vi "Main Engine Path and Folder Info.vi"(8 "error in":errorcluster) -> (0 "error out":errorcluster, 1 "LabVIEW Data":path, 2 "Spare 2":path, 3 "Config":path, 4 "DynData File":path, 5 "Data Logging":path, 7 "TDMS-Logging":path)   [LabVIEW 2024]
doc: "All Rights Reserved © 2017 SyncSols"
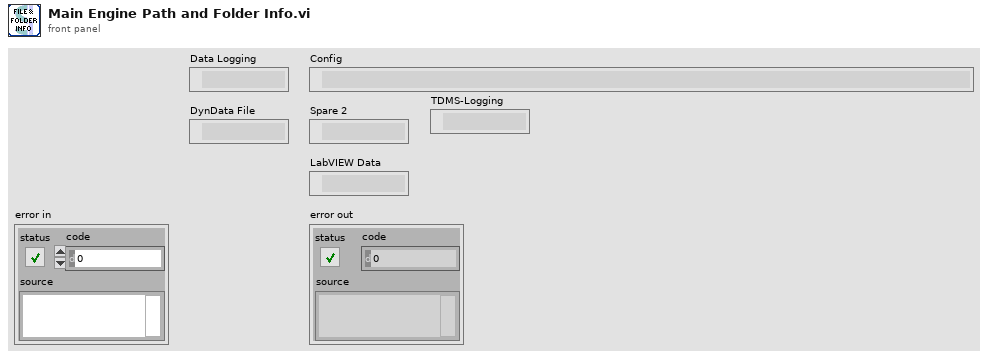
[diagram p1: front panel]
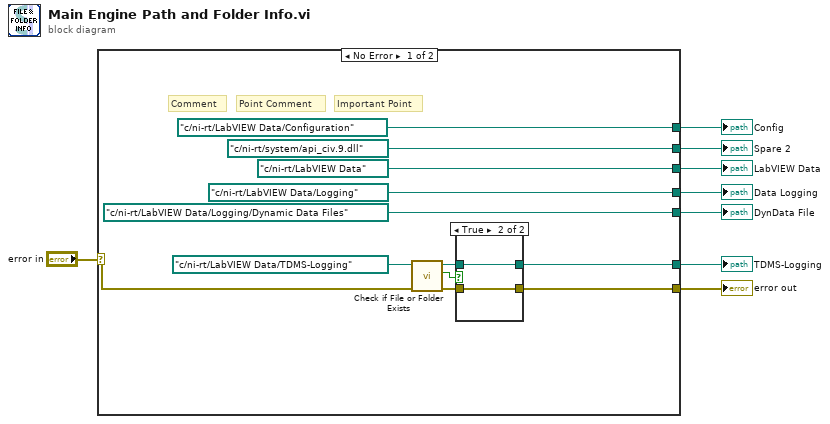
[diagram p0: block diagram]
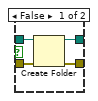
[diagram p2: hidden frame]
diagram:
  n1 = case shown="No Error" "error in" {
    selector: "error in" -> [w14 w27]
    tunnel: [w9 w27] -> w8
    tunnel: [path "c:/ni-rt/LabVIEW Data/Configuration" ("MIL 1553 B") _] -> w6
    tunnel: [path "c:/ni-rt/system/api_civ.9.dll" ("ARNIC 429") _] -> w5
    tunnel: [path "c:/ni-rt/LabVIEW Data" ("Path") _] -> w4
    tunnel: [path "c:/ni-rt/LabVIEW Data/Logging" ("Path") _] -> w3
    tunnel: [path "c:/ni-rt/LabVIEW Data/Logging/Dynamic Data Files" ("Path") _] -> w2
    tunnel: [w10 _] -> w1
    frame No Error {
      # "Important Point"
      # "Point Comment"
      # "Comment"
      n2 = call <vilib>:"Check if File or Folder Exists.vi"("error in (no error)"=w14, "path"=path "c:/ni-rt/LabVIEW Data/TDMS-Logging" ("Path")) -> ("error out"=w11:errorcluster, "file or folder exists?"=w12:bool, "dup path"=w13:path)  [unwired: 7 in]
      n3 = case shown="True" w12 {
        tunnel: w13 -> [w24 w26]
        tunnel: w11 -> [w22 w25]
        tunnel: [w23 w26] -> w10
        tunnel: [w21 w25] -> w9
        frame False {
          n4 = Create Folder(path (use dialog)=w24, error in=w22) -> (created path=w23:path, error out=w21:errorcluster)  [unwired: 1 in, 1 out]
        }
        frame True {
        }
      }
    }
    frame Error {
    }
  }
  "error out" <- w8
  "Config" <- w6
  "Spare 2" <- w5
  "LabVIEW Data" <- w4
  "Data Logging" <- w3
  "DynData File" <- w2
  "TDMS-Logging" <- w1
